vi "Read TCF Data.vi"(8 "error in (no error)":errorcluster, 11 "QPA TCF Parser in":refnum<class "QPA TCF Parser.lvclass">) -> (0 "error out":errorcluster, 2 "TCF Data":T1[](array[typedef]), 3 "QPA TCF Parser out":refnum<class "QPA TCF Parser.lvclass">)   [LabVIEW 2016, in "QPA TCF Parser.lvlib" / "QPA TCF Parser.lvclass"]
uses:
  QPA TCF Parser.lvclass
  Controls/Worksheet Data.ctl
  QPA TCF Parser.lvclass/QPA TCF Parser.ctl
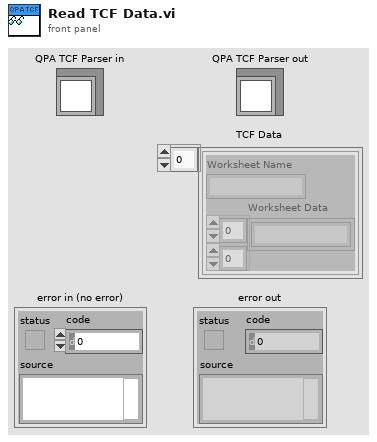
[diagram p1: front panel]
types:
  T1 = typedef "QPA TCF Parser.lvlib/QPA TCF Parser.lvclass/Worksheet Data.ctl" = cluster{"Worksheet Name":string, "Worksheet Data":string[][]}
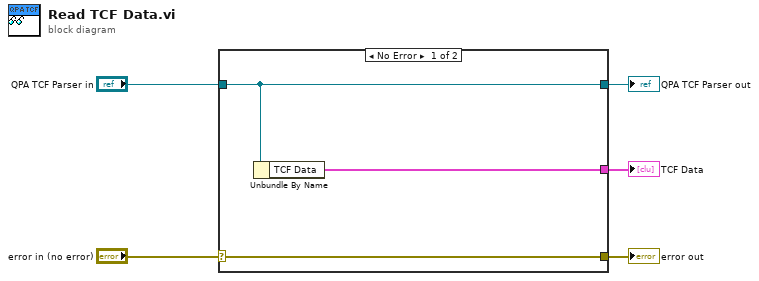
[diagram p0: block diagram]
diagram:
  n1 = case shown="No Error" "error in (no error)" {
    selector: "error in (no error)" -> [w8 w9]
    tunnel: [w8 w9] -> w4
    tunnel: [w7 w10] -> w2
    tunnel: "QPA TCF Parser in" -> [w7 w10]
    tunnel: [w6 _] -> w1
    frame No Error {
      n2 = Unbundle By Name(w7) -> ("TCF Data"=w6:T1[])
    }
    frame Error {
    }
  }
  "error out" <- w4
  "QPA TCF Parser out" <- w2
  "TCF Data" <- w1
